vi "RemoteTester.vi"() -> ()   [LabVIEW 2019]
uses:
  <vilib>/Platform/TimedLoop/XDataNode/timing_clust.ctl
  <vilib>/Platform/TimedLoop/XDataNode/nitl_modes.ctl
  <vilib>/Platform/TimedLoop/XDataNode/wakeup.ctl
  <vilib>/myRIO/Instrument Drivers/Onboard IO/DIO/typedefs/DIO Reference.ctl
  <vilib>/myRIO/Common/Instrument Driver Framework/Utilities/typedefs/myRIO Generic Hardware Reference.ctl
  <vilib>/myRIO/Common/Instrument Driver Framework/Utilities/typedefs/Hardware Version Enum.ctl
  <vilib>/myRIO/Common/Instrument Driver Framework/Utilities/typedefs/myRIO v1.0 Reference.ctl
  <vilib>/myRIO/Common/Instrument Driver Framework/Utilities/typedefs/Generic FPGA Reference.ctl
  <vilib>/myRIO/Common/Instrument Driver Framework/myRIO v1.0/DIO/typedefs/DIO Channels List.ctl
  <vilib>/myRIO/Common/Instrument Driver Framework/myRIO v1.0/DIO/typedefs/DIO Channels Enum.ctl
  <vilib>/userDefined/High Color/nirio_resource_hc.ctl
  <vilib>/myRIO/Common/Instrument Driver Framework/Utilities/vis/Is FPGA Ref Available.vi
  <vilib>/myRIO/Common/Instrument Driver Framework/myRIO v1.0/DIO/vis/myRIO v1.1 Open DIO.vi
  <vilib>/myRIO/Instrument Drivers/Onboard IO/DIO/vis/Write.vi
  <vilib>/myRIO/Common/Instrument Driver Framework/Utilities/vis/Validate Channels.vi
  <vilib>/myRIO/Common/Instrument Driver Framework/myRIO v1.0/DIO/vis/myRIO v1.0 Reserve DIO.vi
  <vilib>/myRIO/Common/Instrument Driver Framework/myRIO v1.0/Resource Manager/vis/myRIO v1.0 Reserve Channel List.vi
  <vilib>/myRIO/Common/Instrument Driver Framework/myRIO v1.0/DIO/vis/myRIO v1.0 Build MUX Configuration DIO.vi
  <vilib>/myRIO/Common/Instrument Driver Framework/myRIO v1.0/Resource Manager/vis/myRIO v1.0 Reserve Channel.vi
  <vilib>/myRIO/Common/Instrument Driver Framework/myRIO v1.0/Resource Manager/vis/myRIO v1.0 Unreserve Channel.vi
  <vilib>/myRIO/Common/Instrument Driver Framework/myRIO v1.0/Resource Manager/vis/myRIO v1.0 Create Configuration List.vi
  <vilib>/myRIO/Common/Instrument Driver Framework/myRIO v1.0/Resource Manager/vis/myRIO v1.0 Build Mutex Name.vi
  <vilib>/rvi/Analysis/host/Private/Sample Rate To Loop Time (ticks).vi
  <vilib>/Utility/error.llb/Error Cluster From Error Code.vi
  <vilib>/rvi/errors/niLvFpgaAdjustHostInterfaceError.vi
  <vilib>/measure/mamon.llb/Trigger Detection for 1 Channel.vi
  <vilib>/measure/matone.llb/Extract Single Tone Information 1 Chan.vi
  <vilib>/FPGAPlugInAG/Dynamic/niLvFpga_Abort_Dynamic.vi
  <vilib>/FPGAPlugInAG/Dynamic/niLvFpga_Close_Dynamic.vi
  <vilib>/Utility/VariantDataType/GetNumericInfo.vi
  <vilib>/myRIO/Common/Instrument Driver Framework/myRIO v1.0/myRIO v1.1 Open.vi
  <vilib>/myRIO/Common/Instrument Driver Framework/Utilities/vis/IO Manager.vi
  <vilib>/myRIO/Common/Instrument Driver Framework/Utilities/vis/Configuration Manager.vi
  <vilib>/myRIO/Common/Instrument Driver Framework/myRIO v1.0/Resource Manager/vis/myRIO v1.0 Configure IO.vi
  <vilib>/myRIO/Common/Instrument Driver Framework/myRIO v1.0/myRIO v1.0 Close.vi
  <vilib>/myRIO/Common/Instrument Driver Framework/myRIO v1.0/DIO/vis/myRIO v1.0 Write DIO.vi
  <vilib>/rvi/interface/nirviMethod/nirviMethod.xnode
  <vilib>/rvi/interface/nirviReadWriteControl/nirviReadWriteControl.xnode
  <vilib>/rvi/interface/nirviCloseFPGA/nirviCloseFPGA.xnode
  <vilib>/platform/TimedLoop/XDataNode/XDataNode.xnode
  <vilib>/myRIO/Express VI/Onboard Devices/LED/LED Express VI.xnode
  <vilib>/myRIO/Instrument Drivers/Onboard IO/DIO/vis/myRIO DIO Open.xnode
  <vilib>/rvi/errors/niLvFpgaMergeErrorWithErrorCode.vi
  <vilib>/rvi/interface/Simulation/niFpgaSimulationCallBeginRW.vi
  NiFpgaLv.dll
  <vilib>/rvi/Analysis/host/Public/NI_FpgaMspHost.lvlib
  <vilib>/FPGAPlugInAG/Dynamic/niLvFpga_ReadFifo_Dynamic.vi
  <vilib>/measure/NI_MAPro.lvlib
  <vilib>/Platform/TimedLoop/XDataNode/XDNodeRunTimeDep.lvlib
  <vilib>/myRIO/Instrument Drivers/Onboard IO/DIO/DIO.lvlib
panel:
  out "aLL":dbl[][](array[numeric])
  in  "LED0":bool
  in  "stop test loop":bool
  out "x-y":dbl=43.60094893016756
  out "Freq":dbl=99.99999999997463
  out "G [um/mA]":dbl=0.0002339690708833829 format="%#_2g"
  in  "stop":bool=TRUE
  in  "MainTab":T1(tab)=enum."Bode Analysis"
  in  "Sine wave properties":T2={"Frequency (periods/tick)"=0.0, "Phase offset (periods)"=0.0, "Scale factor"=0.5, "Amplitude offset"=0.0}
  in  "Sampling Rate":dbl=1024.0 max=100000.0
  in  "Generated Frequency(Hz)":dbl=2000.0
  in  "TimeDataTab":enum32{"Output", "Input", "Triggered Data"}(tab)=enum."Triggered Data"
  out "Output Time Data":dbl[](graph)=[2.0856, 2.0856, 2.0823, 2.0856, 2.0823, 2.0856, 2.0823, 2.0856, 2.0856, 2.0823, 2.0856, 2.0823, 2.0856, 2.0823, 2.0856, 2.0823, 2.0823, 2.0856, 2.0823, 2.0823, 2.0823, 2.0856, 2.0856, 2.0823, 2.0856, 2.0823, 2.0856, 2.0856, 2.0856, 2.0823, 2.0856, 2.0856, 2.0856, 2.0856, 2.0856, 2.0856, 2.0823, 2.0856, 2.0856, 2.0823, 2.0856, 2.0856, 2.0823, 2.0823, 2.0856, 2.0823, 2.0823, 2.0856, 2.0856, 2.0856, 2.0823, 2.0856, 2.0823, 2.0823, 2.0856, 2.0856, 2.0856, 2.0823, 2.0889, 2.0856, 2.0856, 2.0856, 2.0856, 2.0856, 2.0823, 2.0823, 2.0823, 2.0823, 2.0856, 2.0823, 2.0856, 2.079, 2.0856, 2.0823, 2.0823, 2.0856, 2.0823, 2.0823, 2.0823, 2.0856, 2.0823, 2.0856, 2.0856, 2.0856, 2.0856, 2.0823, 2.0856, 2.0823, 2.0856, 2.0856, 2.0823, 2.0856, 2.0823, 2.0856, 2.0823, 2.0856, 2.0856, 2.0823, 2.0856, 2.0856, 2.0856, 2.0823, 2.0856, 2.0856, 2.0823, 2.0856, 2.0856, 2.0856, 2.0823, 2.0856, 2.0856, 2.0856, 2.0856, 2.0856, 2.0856, 2.0823, 2.0856, 2.0889, 2.0823, 2.0856, 2.0823, 2.0856, 2.0823, 2.0856, 2.0856, 2.0823, 2.0856, 2.0823, 2.0856, 2.0823, 2.0856, 2.0823, 2.0823, 2.0856, 2.0823, 2.0856, 2.0823, 2.0856, 2.0856, 2.0856, 2.0856, 2.0823, 2.0856, 2.0823, 2.0856, 2.0823, 2.0856, 2.0856, 2.0823, 2.0856, 2.0856, 2.0856, 2.079, 2.0823, 2.0856, 2.0823, 2.0856, 2.0856, 2.0856, 2.0823, 2.0856, 2.0856, 2.0823, 2.0856, 2.0856, 2.0856, 2.0823, 2.0856, 2.0823, 2.0823, 2.0856, 2.0856, 2.0823, 2.079, 2.0889, 2.0823, 2.0823, 2.0856, 2.0823, 2.0823, 2.0823, 2.0856, 2.0856, 2.0823, 2.0856, 2.0856, 2.0823, 2.0823, 2.0856, 2.0823, 2.0823, 2.0823, 2.0856, 2.0823, 2.079, 2.0889, 2.0823, 2.0823, 2.0856, 2.0856, 2.0823, 2.0823, 2.0856, 2.0823, 2.0823, 2.0856, 2.0856, 2.0856, 2.0823, 2.0889, 2.0856, 2.0856, 2.0856, 2.0856, 2.0856, 2.0823, 2.0823, 2.0823, 2.0823, 2.0856, 2.0823, 2.0856, 2.0823, 2.0856, 2.0823, 2.0889, 2.0823, 2.0823, 2.0856, 2.0823, 2.0823, 2.0823, 2.0889, 2.0823, 2.0823, 2.0889, 2.0823, 2.0856, 2.0823, 2.0889, 2.0856, 2.0856, 2.0889, 2.0823, 2.0823, 2.0823, 2.0856, 2.0823, 2.0823, 2.0823, 2.0856, 2.0823, 2.0823, 2.0856, 2.0823, 2.0823, 2.0856, 2.0823, 2.0823, 2.0823, 2.0889, 2.0823, 2.0823, 2.0856, 2.0856, 2.0856, 2.0823, 2.0856, 2.0823, 2.0856, 2.0856, 2.0823, 2.0823, 2.0856, 2.0856, 2.0823, 2.0823, 2.0856, 2.0823, 2.0856, 2.0823, 2.0856, 2.0823, 2.0856, 2.0856, 2.0823, 2.0856, 2.0823, 2.0856, 2.0856, 2.0823, 2.0856, 2.0856, 2.0856, 2.0856, 2.0856, 2.0823, 2.0856, 2.0823, 2.0823, 2.0856, 2.0823, 2.0856, 2.0823, 2.0856, 2.0823, 2.0823, 2.0856, 2.0823, 2.0823, 2.0823, 2.0856, 2.0823, 2.0856, 2.0856, 2.0856, 2.0823, 2.0823, 2.0889, 2.0823, 2.0823, 2.0856, 2.0856, 2.0823, 2.079, 2.0856, 2.0823, 2.079, 2.0856, 2.0823, 2.0856, 2.079, 2.0856, 2.0823, 2.0823, 2.0823, 2.0856, 2.0856, 2.0856, 2.0889, 2.0823, 2.0856, 2.0856, 2.0856, 2.0823, 2.0823, 2.0856, 2.0823, 2.0856, 2.0823, 2.0856, 2.0823, 2.0823, 2.0856, 2.0823, 2.0856, 2.0823, 2.0856, 2.0856, 2.0823, 2.0856, 2.079, 2.0856, 2.0823, 2.0856, 2.0823, 2.0823, 2.0856, 2.0823, 2.0856, 2.0856, 2.0823, 2.0856, 2.0823, 2.0856, 2.079, 2.0889, 2.0823, 2.0823, 2.0823, 2.0823, 2.0823, 2.0823, 2.0856, 2.079, 2.0856, 2.0823, 2.0823, 2.0856, 2.0823, 2.0856, 2.0823, 2.0823, 2.0856, 2.0823, 2.0856, 2.0856, 2.0856, 2.0856, 2.0856, 2.0856, 2.0823, 2.0856, 2.0823, 2.0889, 2.0823, 2.0889, 2.0856, 2.0823, 2.0856, 2.0823, 2.0823, 2.0823, 2.0856, 2.0823, 2.0823, 2.0889, 2.0823, 2.0889, 2.0823, 2.0856, 2.0823, 2.0823, 2.0856, 2.0823, 2.0856, 2.0823, 2.0856, 2.0823, 2.0823, 2.0856, 2.0823, 2.0823, 2.0823, 2.0856, 2.0823, 2.0856, 2.0856, 2.0856, 2.0823, 2.0856, 2.0856, 2.0823, 2.0823, 2.0856, 2.0823, 2.0823, 2.0823, 2.0856, 2.0823, 2.0856, 2.0823, 2.0823, 2.0823, 2.0823, 2.0856, 2.079, 2.0856, 2.0856, 2.0823, 2.0856, 2.0856, 2.0856, 2.0823, 2.0856, 2.0856, 2.0823, 2.0856, 2.0856, 2.0856, 2.0823, 2.0856, 2.0856, 2.0823, 2.079, 2.0856, 2.0856, 2.0823, 2.0856, 2.0856, 2.0856, 2.0856, 2.0823, 2.0889, 2.0823, 2.0856, 2.0856, 2.0823, 2.0856, 2.0823, 2.0856, 2.079, 2.0856, 2.0823, 2.0823, 2.0856, 2.0856, 2.0823, 2.079, 2.0823, 2.0823, 2.0823, 2.0856, 2.0823, 2.0823, 2.0823, 2.0856, 2.0823, 2.0823, 2.0823, 2.0856, 2.0823, 2.0823, 2.0823, 2.0823, 2.0856, 2.0856, 2.0856, 2.0856, 2.0856, 2.0856, 2.0823, 2.0856, 2.0856, 2.0823, 2.0856, 2.0856, 2.0889, 2.0823, 2.0889, 2.0856, 2.0823, 2.0856, 2.0856, 2.0823, 2.079, 2.0856, 2.0856, 2.0823, 2.0856, 2.0856, 2.0856, 2.079, 2.0889, 2.0823, 2.0856, 2.0856, 2.0856, 2.0856, 2.079, 2.0889, 2.0856, 2.0856, 2.0856, 2.0856, 2.0856, 2.079, 2.0889, 2.079, 2.0823, 2.0856, 2.0856, 2.0823, 2.0823, 2.0889, 2.0823, 2.0823, 2.0856, 2.0823, 2.0823, 2.0823, 2.0856, 2.0823, 2.0823, 2.0856, 2.0823, 2.0856, 2.0823, 2.0856, 2.0823, 2.0823, 2.0856, 2.0823, 2.0856, 2.0823, 2.0889, 2.079, 2.0823, 2.0856, 2.0823, 2.0856, 2.0856, 2.0889, 2.0823, 2.0856, 2.0856, 2.0823, 2.0823, 2.0823, 2.0856, 2.079, 2.0856, 2.0856, 2.0856, 2.0823, 2.0823, 2.0856, 2.0823, 2.0856, 2.0823, 2.0856, 2.0823, 2.0823, 2.0856, 2.0856, 2.0889, 2.0823, 2.0856, 2.0856, 2.0823, 2.0823, 2.0823, 2.0856, 2.0823, 2.0856, 2.0856, 2.0823, 2.0856, 2.0823, 2.0856, 2.079, 2.0856, 2.0856, 2.0823, 2.0856, 2.0823, 2.0856, 2.0823, 2.0823, 2.0856, 2.0823, 2.0889, 2.0823, 2.0856, 2.0823, 2.0856, 2.0856, 2.0823, 2.0856, 2.0823, 2.0856, 2.0823, 2.0856, 2.0856, 2.0823, 2.0856, 2.0856, 2.0856, 2.0823, 2.0856, 2.0856, 2.0823, 2.0856, 2.0856, 2.0889, 2.0823, 2.0856, 2.0856, 2.0823, 2.0823, 2.0856, 2.0856, 2.079, 2.0856, 2.0856, 2.0823, 2.0856, 2.0823, 2.0856, 2.0823, 2.0856, 2.079, 2.0856, 2.0856, 2.0823, 2.0856, 2.0823, 2.0856, 2.0823, 2.0823, 2.0856, 2.0823, 2.0823, 2.0823, 2.0856, 2.0823, 2.0856, 2.0856, 2.0823, 2.0856, 2.0823, 2.0856, 2.0823, 2.0856, 2.0856, 2.0823, 2.0823, 2.0856, 2.0889, 2.0823, 2.0856, 2.0889, 2.0823, 2.0856, 2.0823, 2.0856, 2.0823, 2.0856, 2.0889, 2.0823, 2.0856, 2.0823, 2.0889, 2.0823, 2.0856, 2.0856, 2.0823, 2.0823, 2.0856, 2.0856, 2.079, 2.0856, 2.0856, 2.0856, 2.0823, 2.0823, 2.0823, 2.0856, 2.0856, 2.0856, 2.0856, 2.0856, 2.0856, 2.0856, 2.0856, 2.0856, 2.0823, 2.0823, 2.0856, 2.0823, 2.0823, 2.0823, 2.0856, 2.079, 2.0823, 2.0856, 2.0823, 2.0823, 2.0823, 2.0889, 2.079, 2.0856, 2.0856, 2.0823, 2.0823, 2.0823, 2.0889, 2.079, 2.0823, 2.0856, 2.0823, 2.0856, 2.0856, 2.0889, 2.0823, 2.0856, 2.0856, 2.0823, 2.0856, 2.0823, 2.0856, 2.0823, 2.0856, 2.0823, 2.0856, 2.0856, 2.0823, 2.0889, 2.0823, 2.0856, 2.0823, 2.0823, 2.0856, 2.0823, 2.0856, 2.0823, 2.0823, 2.0823, 2.0823, 2.0856, 2.0856, 2.0823, 2.0823, 2.0856, 2.0823, 2.0823, 2.0856, 2.079, 2.0823, 2.0823, 2.0856, 2.0823, 2.0823, 2.0856, 2.0856, 2.0823, 2.0823, 2.0856, 2.0823, 2.0823, 2.0856, 2.0856, 2.0856, 2.0823, 2.0889, 2.0823, 2.0823, 2.0823, 2.0856, 2.0856, 2.0856, 2.0889, 2.0823, 2.0856, 2.0823, 2.0856, 2.0823, 2.0856, 2.0856, 2.0823, 2.0856, 2.0856, 2.0856, 2.0823, 2.0823, 2.0856, 2.0823, 2.0856, 2.0823, 2.0823, 2.0823, 2.0823, 2.0889, 2.0823, 2.0856, 2.0823, 2.0856, 2.0823, 2.0823, 2.0856, 2.0823, 2.0856, 2.0823, 2.0823, 2.0823, 2.0823, 2.0856, 2.0856, 2.0856, 2.0823, 2.0823, 2.0856, 2.0823, 2.0856, 2.0823, 2.0856, 2.0823, 2.0889, 2.0856, 2.0823, 2.0823, 2.0823, 2.0856, 2.079, 2.0856, 2.0856, 2.0823, 2.0856, 2.0856, 2.0856, 2.079, 2.0823, 2.0856, 2.0823, 2.0823, 2.0856, 2.0856, 2.0823, 2.0889, 2.0856, 2.0823, 2.0823, 2.0856, 2.0856, 2.0823, 2.0889, 2.0856, 2.0856, 2.0856, 2.0823, 2.0856, 2.0823, 2.0856, 2.0856, 2.0823, 2.0856, 2.0856, 2.0856, 2.0823, 2.0856, 2.0856, 2.0823, 2.0856, 2.0823, 2.0856, 2.0823, 2.0856, 2.0823, 2.079, 2.0856, 2.0823, 2.0856, 2.0823, 2.0889, 2.0823, 2.0856, 2.0823, 2.0823, 2.0856, 2.0823, 2.0856, 2.079, 2.0856, 2.0856, 2.0823, 2.0856, 2.0823, 2.0856, 2.0823, 2.0856, 2.0856, 2.0823, 2.0856, 2.0856, 2.0856, 2.0856, 2.0856, 2.0856, 2.079, 2.0856, 2.0823, 2.0856, 2.079, 2.0856, 2.0889, 2.0856, 2.0856, 2.0823, 2.0856, 2.079, 2.0856, 2.0856, 2.0823, 2.0856, 2.0856, 2.0889, 2.0823, 2.0856, 2.0823, 2.0823, 2.0856, 2.0823, 2.0856, 2.0823, 2.0856, 2.0856, 2.0856, 2.0856, 2.0823, 2.0823, 2.0823, 2.0856, 2.0823, 2.0823, 2.0856, 2.0823, 2.0823, 2.0823, 2.0856, 2.079, 2.0823, 2.0856, 2.0856, 2.0823, 2.079, 2.0856, 2.0823, 2.0823, 2.0856, 2.0823, 2.0856, 2.0856, 2.0889, 2.0856, 2.0856, 2.0856, 2.0823, 2.0823, 2.0823, 2.0856, 2.0823, 2.0856, 2.0856, 2.0856]
  out "InputTimeData":dbl[](graph)=[6.5538, 6.7485, 6.6594, 6.3096, 5.7222, 4.8609, 3.9567, 3.0294, 2.1252, 1.2012, 0.5808, 0.165, 0.0, 0.132, 0.5148, 1.1088, 2.0097, 2.904, 3.8544, 4.7487, 5.6496, 6.2436, 6.6297, 6.7584, 6.5868, 6.1776, 5.5572, 4.6331999999999995, 3.729, 2.7786, 1.8975, 1.0197, 0.4488, 0.0957, 0.009899999999999999, 0.2112, 0.6534, 1.3002, 2.2407, 3.1515, 4.0986, 5.082, 5.8278, 6.369, 6.6857999999999995, 6.7386, 6.5076, 6.0324, 5.3592, 4.4022, 3.4848, 2.5377, 1.5708, 0.8481, 0.3333, 0.0495, 0.0363, 0.297, 0.8052, 1.6071, 2.4783, 3.399, 4.3395, 5.2932, 5.9928, 6.4746, 6.7254, 6.699, 6.4086, 5.8674, 5.0424, 4.158, 3.234, 2.3199, 1.3662, 0.6897, 0.2343, 0.0165, 0.0825, 0.4092, 0.9768, 1.8215999999999999, 2.7192, 3.6498, 4.5573, 5.4912, 6.1314, 6.567, 6.7584, 6.6462, 6.2898, 5.6958, 4.8246, 3.9138, 2.9865, 2.0856, 1.1715, 0.5577, 0.1518, 0.0, 0.1452, 0.5346, 1.1418, 2.046, 2.9634, 3.894, 4.785, 5.6793, 6.2667, 6.6396, 6.7551, 6.5736, 6.1545, 5.5241999999999996, 4.5936, 3.6894, 2.739, 1.7489999999999999, 0.99, 0.429, 0.0858, 0.0132, 0.2244, 0.6798, 1.3332, 2.2803, 3.1944, 4.1382, 5.115, 5.8542, 6.3888, 6.699, 6.732, 6.4845, 6.006, 5.2041, 4.3626, 3.4419, 2.4981, 1.5378, 0.8184, 0.31679999999999997, 0.0429, 0.0429, 0.31679999999999997, 0.8316, 1.6434, 2.5179, 3.4419, 4.3824, 5.3262, 6.0192, 6.4944, 6.732, 6.6924, 6.3888, 5.841, 5.0094, 4.1184, 3.1944, 2.2605, 1.3332, 0.6666, 0.2178, 0.0033, 0.0924, 0.429, 1.0032, 1.8612, 2.7588, 3.6894, 4.5936, 5.5241999999999996, 6.1545, 6.5802, 6.7584, 6.6363, 6.2667, 5.6628, 4.785, 3.8742, 2.9436, 1.914, 1.1418, 0.5346, 0.1386, 0.0, 0.15839999999999999, 0.5577, 1.188, 2.0856, 3.0063, 3.9369, 4.9533, 5.709, 6.2898, 6.6528, 6.7518, 6.5604, 6.1314, 5.4912, 4.5573, 3.6498, 2.6994, 1.6962, 0.9603, 0.4092, 0.07919999999999999, 0.0165, 0.2409, 0.7029, 1.485, 2.3199, 3.234, 4.1778, 5.1513, 5.8806, 6.4086, 6.7056, 6.7254, 6.468, 5.9796, 5.1678, 4.3197, 3.399, 2.4585, 1.5015, 0.792, 0.297, 0.0363, 0.0495, 0.3333, 0.8613, 1.6962, 2.5575, 3.4848, 4.4187, 5.3592, 6.0456, 6.5076, 6.7518, 6.6857999999999995, 6.369, 5.8145999999999995, 4.9698, 4.0788, 3.1515, 2.2209, 1.3002, 0.6402, 0.2046, 0.0, 0.099, 0.4488, 1.0362, 1.8975, 2.8017, 3.729, 4.7652, 5.5572, 6.1908, 6.5934, 6.7584, 6.6264, 6.2436, 5.6331, 4.7487, 3.8346, 2.904, 1.8777, 1.1088, 0.5148, 0.1287, 0.0, 0.1716, 0.5808, 1.221, 2.1252, 3.0492, 3.9798, 4.9896, 5.7387, 6.3096, 6.6627, 6.7485, 6.5472, 6.1049999999999995, 5.3427, 4.5177, 3.5871, 2.6598, 1.6599, 0.9306, 0.3894, 0.0693, 0.019799999999999998, 0.2574, 0.726, 1.518, 2.3562, 3.2736, 4.2207, 5.1876, 5.9103, 6.4251, 6.732, 6.7221, 6.4515, 5.9532, 5.1348, 4.2801, 3.3594, 2.4189, 1.4652, 0.7656, 0.2838, 0.0132, 0.0594, 0.363, 0.891, 1.7292, 2.6004, 3.5244, 4.4583, 5.3922, 6.0687, 6.5241, 6.7518, 6.6759, 6.3492, 5.7816, 4.9368, 4.0392, 3.1086, 2.0658, 1.2671999999999999, 0.6171, 0.1914, 0.0, 0.1122, 0.4686, 1.0626, 1.9338, 2.8446, 3.7719, 4.8048, 5.5869, 6.2106, 6.6066, 6.7584, 6.6132, 6.2238, 5.6034, 4.7124, 3.795, 2.8644, 1.8414, 1.0791, 0.49169999999999997, 0.1188, 0.0066, 0.1848, 0.6039, 1.3497, 2.1648, 3.0888, 4.0194, 5.0292, 5.7684, 6.3294, 6.6726, 6.7452, 6.534, 6.0786, 5.3064, 4.4781, 3.5442, 2.6202, 1.6236, 0.9042, 0.3696, 0.039599999999999996, 0.0264, 0.2739, 0.7524, 1.5543, 2.3958, 3.3165, 4.2603, 5.2404, 5.94, 6.4416, 6.7353, 6.7155, 6.435, 5.9268, 5.0985, 4.2405, 3.3165, 2.376, 1.4322, 0.7392, 0.264, 0.0132, 0.066, 0.3795, 0.9174, 1.7688, 2.64, 3.564, 4.6134, 5.4252, 6.0918, 6.5405999999999995, 6.7551, 6.666, 6.3294, 5.7552, 4.8807, 3.9996, 3.069, 2.0295, 1.2342, 0.594, 0.1782, 0.0, 0.1221, 0.49169999999999997, 1.188, 1.9734, 2.8842, 3.8148, 4.8444, 5.6166, 6.2337, 6.6198, 6.7584, 6.6, 6.2007, 5.4747, 4.6728, 3.7521, 2.8215, 1.8051, 1.0493999999999999, 0.462, 0.1056, 0.0066, 0.198, 0.627, 1.3827, 2.2011, 3.1284, 4.059, 5.0622, 5.7981, 6.3492, 6.7056, 6.7419, 6.5175, 6.0555, 5.2734, 4.4385, 3.5046, 2.5806, 1.5906, 0.8778, 0.3498, 0.033, 0.033, 0.2904, 0.7788, 1.5906, 2.4387, 3.3792, 4.2999, 5.2734, 5.9664, 6.4614, 6.7386, 6.7089, 6.4152, 5.8971, 5.0622, 4.2009, 3.2736, 2.2209, 1.3992, 0.7128, 0.2508, 0.0066, 0.0726, 0.3993, 0.9438, 1.8051, 2.6796, 3.6069, 4.653, 5.4582, 6.1182, 6.5538, 6.7584, 6.6594, 6.2964, 5.6331, 4.8444, 3.9567, 3.0294, 1.9932, 1.2012, 0.5676, 0.165, 0.0, 0.132, 0.5148, 1.221, 2.0097, 2.9238, 3.8544, 4.8807, 5.6496, 6.2568, 6.6297, 6.7551, 6.5868, 6.1776, 5.4417, 4.6331999999999995, 3.7092, 2.7786, 1.7688, 1.0197, 0.4389, 0.0693, 0.0132, 0.2112, 0.6534, 1.4157, 2.2407, 3.1713, 4.0986, 5.0985, 5.8278, 6.369, 6.7122, 6.7353, 6.501, 6.0324, 5.2404, 4.4022, 3.4617, 2.4189, 1.5543, 0.8481, 0.3333, 0.0264, 0.0363, 0.3069, 0.8052, 1.6236, 2.4783, 3.4188, 4.4583, 5.3064, 5.9928, 6.4746, 6.7452, 6.699, 6.3953999999999995, 5.8674, 5.0292, 4.158, 3.234, 2.1846, 1.3497, 0.6897, 0.2343, 0.0066, 0.0825, 0.4191, 1.0626, 1.8414, 2.7192, 3.6498, 4.6926, 5.4912, 6.1413, 6.567, 6.7584, 6.6462, 6.2766, 5.6034, 4.8048, 3.9138, 2.9865, 1.9536, 1.1715, 0.5478, 0.1518, 0.0, 0.1452, 0.5346, 1.254, 2.0658, 2.9634, 3.894, 4.917, 5.6793, 6.2766, 6.6726, 6.7518, 6.5736, 6.1545, 5.4087, 4.5936, 3.6696, 2.739, 1.7292, 0.99, 0.4191, 0.0594, 0.0132, 0.2244, 0.6798, 1.452, 2.2803, 3.2142, 4.2603, 5.1348, 5.8542, 6.3953999999999995, 6.7188, 6.732, 6.4845, 6.006, 5.2041, 4.3626, 3.4188, 2.376, 1.518, 0.8184, 0.31679999999999997, 0.0231, 0.0429, 0.3234, 0.8316, 1.6599, 2.5179, 3.4617, 4.4979, 5.3427, 6.0192, 6.4944, 6.7452, 6.6924, 6.3789, 5.7552, 4.9896, 4.1184, 3.1713, 2.145, 1.3167, 0.6666, 0.2178, 0.0033, 0.0924, 0.4389, 1.0956, 1.8777, 2.7588, 3.6894, 4.7289, 5.5241999999999996, 6.1644, 6.6264, 6.7584, 6.6363, 6.2568, 5.5704, 4.7652, 3.8742, 2.9436, 1.914, 1.1418, 0.5246999999999999, 0.1056, 0.0, 0.15839999999999999, 0.5676, 1.2837, 2.1054, 3.0063, 3.9369, 4.9533, 5.709, 6.2964, 6.6792, 6.7518, 6.5604, 6.1314, 5.3757, 4.5573, 3.63, 2.5575, 1.6962, 0.9603, 0.3993, 0.0528, 0.019799999999999998, 0.2409, 0.7029, 1.485, 2.3199, 3.2538, 4.2999, 5.1678, 5.8806, 6.4152, 6.7254, 6.7254, 6.468, 5.9796, 5.1678, 4.3197, 3.3792, 2.3397, 1.485, 0.792, 0.297, 0.019799999999999998, 0.0528, 0.3432, 0.9603, 1.6962, 2.5575, 3.5046, 4.5375, 5.3757, 6.0456, 6.5076, 6.7518, 6.6857999999999995, 6.3591, 5.7222, 4.9533, 4.0788, 3.1284, 2.1054, 1.2837, 0.6402, 0.15839999999999999, 0.0, 0.099, 0.462, 1.1253, 1.914, 2.8017, 3.729, 4.7652, 5.5704, 6.1908, 6.6363, 6.7584, 6.6264, 6.2337, 5.5374, 4.7289, 3.8346, 2.904, 1.8777, 1.1088, 0.5016, 0.0957, 0.0033, 0.1716, 0.594, 1.3167, 2.145, 3.0492, 4.1184, 4.9896, 5.7387, 6.3195, 6.6891, 6.7452, 6.5472, 6.1049999999999995, 5.3427, 4.4979, 3.5871, 2.5179, 1.6599, 0.9306, 0.3795, 0.0462, 0.0231, 0.2574, 0.8184, 1.518, 2.3562, 3.2967, 4.3395, 5.2041, 5.9103, 6.435, 6.732, 6.7188, 6.4515, 5.8542, 5.1348, 4.2801, 3.3396, 2.3001, 1.452, 0.7656, 0.2739, 0.0132, 0.0594, 0.363, 0.99, 1.7292, 2.6004, 3.5442, 4.5738, 5.4087, 6.0687, 6.5736, 6.7518, 6.6759, 6.3393, 5.6958, 4.917, 4.0392, 3.0888, 2.0658, 1.254, 0.6171, 0.1452, 0.0, 0.1122, 0.4818, 1.155, 1.9536, 2.8446, 3.795, 4.8048, 5.6034, 6.2106, 6.6462, 6.7584, 6.6132, 6.2106, 5.5044, 4.6926, 3.795, 2.7192, 1.8414, 1.0791, 0.4818, 0.0825, 0.0066, 0.1848, 0.6171, 1.3497, 2.1846, 3.0888, 4.158, 5.0292, 5.7684, 6.3393, 6.699, 6.7452, 6.534, 5.9928, 5.3064, 4.4583, 3.5442, 2.4783, 1.6236, 0.9042, 0.363, 0.039599999999999996, 0.0264, 0.2739, 0.8481, 1.5543, 2.3958, 3.3396, 4.4022, 5.2404, 5.94, 6.4515, 6.7353, 6.7122, 6.435, 5.8278, 5.0985, 4.2405, 3.2967, 2.2605, 1.4157, 0.7392, 0.2112, 0.0132, 0.0693, 0.3795, 1.0197, 1.7688, 2.64, 3.5871, 4.6134, 5.4417, 6.0918, 6.5868, 6.7551, 6.666, 6.3195, 5.6496, 4.8807, 3.9996, 2.9238, 2.0295, 1.221, 0.594, 0.132, 0.0, 0.1221, 0.5016, 1.188, 1.9932, 2.8842, 3.9567, 4.8444, 5.6331, 6.2337, 6.6594, 6.7584, 6.6, 6.1908, 5.4747, 4.653, 3.7521, 2.6796, 1.8051, 1.0362, 0.462, 0.0726, 0.0066, 0.198, 0.7128, 1.3827, 2.2209, 3.1284, 4.2009, 5.0622, 5.7981, 6.3591, 6.7056, 6.7386, 6.5175, 5.9664, 5.2734, 4.4187, 3.5046, 2.4387, 1.5906, 0.8778, 0.3432, 0.033, 0.033, 0.2904, 0.8778, 1.5906, 2.4585, 3.3792, 4.4385, 5.2734, 5.9664, 6.5175, 6.7386, 6.7056, 6.4152, 5.7981, 5.0622, 4.2009, 3.2538, 2.2209, 1.3827, 0.7128, 0.198, 0.0066, 0.07919999999999999, 0.3993, 1.0493999999999999, 1.8051, 2.6796, 3.7521, 4.653, 5.4747, 6.1182, 6.6, 6.7584, 6.6528, 6.2964, 5.6166, 4.8444, 3.9567, 2.8842, 1.9932, 1.188, 0.5676, 0.1221, 0.0, 0.132, 0.5246999999999999, 1.221, 2.0295, 2.9238, 3.9996, 4.8807, 5.6628, 6.2568, 6.666, 6.7551]
  out "Waveform Graph 2":dbl[][](graph)=[[2.0097, 2.904, 3.8544, 4.7487, 5.6496, 6.2436, 6.6297, 6.7584, 6.5868, 6.1776, 5.5572, 4.6331999999999995, 3.729, 2.7786, 1.8975, 1.0197, 0.4488, 0.0957, 0.009899999999999999, 0.2112, 0.6534, 1.3002, 2.2407, 3.1515, 4.0986, 5.082, 5.8278, 6.369, 6.6857999999999995, 6.7386, 6.5076, 6.0324, 5.3592, 4.4022, 3.4848, 2.5377, 1.5708, 0.8481, 0.3333, 0.0495, 0.0363, 0.297, 0.8052, 1.6071, 2.4783, 3.399, 4.3395, 5.2932, 5.9928, 6.4746, 6.7254, 6.699, 6.4086, 5.8674, 5.0424, 4.158, 3.234, 2.3199, 1.3662, 0.6897, 0.2343, 0.0165, 0.0825, 0.4092, 0.9768, 1.8215999999999999, 2.7192, 3.6498, 4.5573, 5.4912, 6.1314, 6.567, 6.7584, 6.6462, 6.2898, 5.6958, 4.8246, 3.9138, 2.9865, 2.0856, 1.1715, 0.5577, 0.1518, 0.0, 0.1452, 0.5346, 1.1418, 2.046, 2.9634, 3.894, 4.785, 5.6793, 6.2667, 6.6396, 6.7551, 6.5736, 6.1545, 5.5241999999999996, 4.5936, 3.6894, 2.739, 1.7489999999999999, 0.99, 0.429, 0.0858, 0.0132, 0.2244, 0.6798, 1.3332, 2.2803, 3.1944, 4.1382, 5.115, 5.8542, 6.3888, 6.699, 6.732, 6.4845, 6.006, 5.2041, 4.3626, 3.4419, 2.4981, 1.5378, 0.8184, 0.31679999999999997, 0.0429, 0.0429, 0.31679999999999997, 0.8316, 1.6434, 2.5179, 3.4419, 4.3824, 5.3262, 6.0192, 6.4944, 6.732, 6.6924, 6.3888, 5.841, 5.0094, 4.1184, 3.1944, 2.2605, 1.3332, 0.6666, 0.2178, 0.0033, 0.0924, 0.429, 1.0032, 1.8612, 2.7588, 3.6894, 4.5936, 5.5241999999999996, 6.1545, 6.5802, 6.7584, 6.6363, 6.2667, 5.6628, 4.785, 3.8742, 2.9436, 1.914, 1.1418, 0.5346, 0.1386, 0.0, 0.15839999999999999, 0.5577, 1.188, 2.0856, 3.0063, 3.9369, 4.9533, 5.709, 6.2898, 6.6528, 6.7518, 6.5604, 6.1314, 5.4912, 4.5573, 3.6498, 2.6994, 1.6962, 0.9603, 0.4092, 0.07919999999999999, 0.0165, 0.2409, 0.7029, 1.485, 2.3199, 3.234, 4.1778, 5.1513, 5.8806, 6.4086, 6.7056, 6.7254, 6.468, 5.9796, 5.1678, 4.3197, 3.399, 2.4585, 1.5015, 0.792, 0.297, 0.0363, 0.0495, 0.3333, 0.8613, 1.6962, 2.5575, 3.4848, 4.4187, 5.3592, 6.0456, 6.5076, 6.7518, 6.6857999999999995, 6.369, 5.8145999999999995, 4.9698, 4.0788, 3.1515, 2.2209, 1.3002, 0.6402, 0.2046, 0.0, 0.099, 0.4488, 1.0362, 1.8975, 2.8017, 3.729, 4.7652, 5.5572, 6.1908, 6.5934, 6.7584, 6.6264, 6.2436, 5.6331, 4.7487, 3.8346, 2.904, 1.8777, 1.1088, 0.5148, 0.1287, 0.0, 0.1716, 0.5808, 1.221, 2.1252, 3.0492, 3.9798, 4.9896, 5.7387, 6.3096, 6.6627, 6.7485, 6.5472, 6.1049999999999995, 5.3427, 4.5177, 3.5871, 2.6598, 1.6599, 0.9306, 0.3894, 0.0693, 0.019799999999999998, 0.2574, 0.726, 1.518, 2.3562, 3.2736, 4.2207, 5.1876, 5.9103, 6.4251, 6.732, 6.7221, 6.4515, 5.9532, 5.1348, 4.2801, 3.3594, 2.4189, 1.4652, 0.7656, 0.2838, 0.0132, 0.0594, 0.363, 0.891, 1.7292, 2.6004, 3.5244, 4.4583, 5.3922, 6.0687, 6.5241, 6.7518, 6.6759, 6.3492, 5.7816, 4.9368, 4.0392, 3.1086, 2.0658, 1.2671999999999999, 0.6171, 0.1914, 0.0, 0.1122, 0.4686, 1.0626, 1.9338, 2.8446, 3.7719, 4.8048, 5.5869, 6.2106, 6.6066, 6.7584, 6.6132, 6.2238, 5.6034, 4.7124, 3.795, 2.8644, 1.8414, 1.0791, 0.49169999999999997, 0.1188, 0.0066, 0.1848, 0.6039, 1.3497, 2.1648, 3.0888, 4.0194, 5.0292, 5.7684, 6.3294, 6.6726, 6.7452, 6.534, 6.0786, 5.3064, 4.4781, 3.5442, 2.6202, 1.6236, 0.9042, 0.3696, 0.039599999999999996, 0.0264, 0.2739, 0.7524, 1.5543, 2.3958, 3.3165, 4.2603, 5.2404, 5.94, 6.4416, 6.7353, 6.7155, 6.435, 5.9268, 5.0985, 4.2405, 3.3165, 2.376, 1.4322, 0.7392, 0.264, 0.0132, 0.066, 0.3795, 0.9174, 1.7688, 2.64, 3.564, 4.6134, 5.4252, 6.0918, 6.5405999999999995, 6.7551, 6.666, 6.3294, 5.7552, 4.8807, 3.9996, 3.069, 2.0295, 1.2342, 0.594, 0.1782, 0.0, 0.1221, 0.49169999999999997, 1.188, 1.9734, 2.8842, 3.8148, 4.8444, 5.6166, 6.2337, 6.6198, 6.7584, 6.6, 6.2007, 5.4747, 4.6728, 3.7521, 2.8215, 1.8051, 1.0493999999999999, 0.462, 0.1056, 0.0066, 0.198, 0.627, 1.3827, 2.2011, 3.1284, 4.059, 5.0622, 5.7981, 6.3492, 6.7056, 6.7419, 6.5175, 6.0555, 5.2734, 4.4385, 3.5046, 2.5806, 1.5906, 0.8778, 0.3498, 0.033, 0.033, 0.2904, 0.7788, 1.5906, 2.4387, 3.3792, 4.2999, 5.2734, 5.9664, 6.4614, 6.7386, 6.7089, 6.4152, 5.8971, 5.0622, 4.2009, 3.2736, 2.2209, 1.3992, 0.7128, 0.2508, 0.0066, 0.0726, 0.3993, 0.9438, 1.8051, 2.6796, 3.6069, 4.653, 5.4582, 6.1182, 6.5538, 6.7584, 6.6594, 6.2964, 5.6331, 4.8444, 3.9567, 3.0294, 1.9932, 1.2012, 0.5676, 0.165, 0.0, 0.132, 0.5148, 1.221, 2.0097, 2.9238, 3.8544, 4.8807, 5.6496, 6.2568, 6.6297, 6.7551, 6.5868, 6.1776, 5.4417, 4.6331999999999995, 3.7092, 2.7786, 1.7688, 1.0197, 0.4389, 0.0693, 0.0132, 0.2112, 0.6534, 1.4157, 2.2407, 3.1713, 4.0986, 5.0985, 5.8278, 6.369, 6.7122, 6.7353, 6.501, 6.0324, 5.2404, 4.4022, 3.4617, 2.4189, 1.5543, 0.8481, 0.3333, 0.0264, 0.0363, 0.3069, 0.8052, 1.6236, 2.4783, 3.4188, 4.4583, 5.3064, 5.9928, 6.4746, 6.7452, 6.699, 6.3953999999999995, 5.8674, 5.0292, 4.158, 3.234, 2.1846, 1.3497, 0.6897, 0.2343, 0.0066, 0.0825, 0.4191, 1.0626, 1.8414, 2.7192, 3.6498, 4.6926, 5.4912, 6.1413, 6.567, 6.7584, 6.6462, 6.2766, 5.6034, 4.8048, 3.9138, 2.9865, 1.9536, 1.1715, 0.5478, 0.1518, 0.0, 0.1452, 0.5346, 1.254, 2.0658, 2.9634, 3.894, 4.917, 5.6793, 6.2766, 6.6726, 6.7518, 6.5736, 6.1545, 5.4087, 4.5936, 3.6696, 2.739, 1.7292, 0.99, 0.4191, 0.0594, 0.0132, 0.2244, 0.6798, 1.452, 2.2803, 3.2142, 4.2603, 5.1348, 5.8542, 6.3953999999999995, 6.7188, 6.732, 6.4845, 6.006, 5.2041, 4.3626, 3.4188, 2.376, 1.518, 0.8184, 0.31679999999999997, 0.0231, 0.0429, 0.3234, 0.8316, 1.6599, 2.5179, 3.4617, 4.4979, 5.3427, 6.0192, 6.4944, 6.7452, 6.6924, 6.3789, 5.7552, 4.9896, 4.1184, 3.1713, 2.145, 1.3167, 0.6666, 0.2178, 0.0033, 0.0924, 0.4389, 1.0956, 1.8777, 2.7588, 3.6894, 4.7289, 5.5241999999999996, 6.1644, 6.6264, 6.7584, 6.6363, 6.2568, 5.5704, 4.7652, 3.8742, 2.9436, 1.914, 1.1418, 0.5246999999999999, 0.1056, 0.0, 0.15839999999999999, 0.5676, 1.2837, 2.1054, 3.0063, 3.9369, 4.9533, 5.709, 6.2964, 6.6792, 6.7518, 6.5604, 6.1314, 5.3757, 4.5573, 3.63, 2.5575, 1.6962, 0.9603, 0.3993, 0.0528, 0.019799999999999998, 0.2409, 0.7029, 1.485, 2.3199, 3.2538, 4.2999, 5.1678, 5.8806, 6.4152, 6.7254, 6.7254, 6.468, 5.9796, 5.1678, 4.3197, 3.3792, 2.3397, 1.485, 0.792, 0.297, 0.019799999999999998, 0.0528, 0.3432, 0.9603, 1.6962, 2.5575, 3.5046, 4.5375, 5.3757, 6.0456, 6.5076, 6.7518, 6.6857999999999995, 6.3591, 5.7222, 4.9533, 4.0788, 3.1284, 2.1054, 1.2837, 0.6402, 0.15839999999999999, 0.0, 0.099, 0.462, 1.1253, 1.914, 2.8017, 3.729, 4.7652, 5.5704, 6.1908, 6.6363, 6.7584, 6.6264, 6.2337, 5.5374, 4.7289, 3.8346, 2.904, 1.8777, 1.1088, 0.5016, 0.0957, 0.0033, 0.1716, 0.594, 1.3167, 2.145, 3.0492, 4.1184, 4.9896, 5.7387, 6.3195, 6.6891, 6.7452, 6.5472, 6.1049999999999995, 5.3427, 4.4979, 3.5871, 2.5179, 1.6599, 0.9306, 0.3795, 0.0462, 0.0231, 0.2574, 0.8184, 1.518, 2.3562, 3.2967, 4.3395, 5.2041, 5.9103, 6.435, 6.732, 6.7188, 6.4515, 5.8542, 5.1348, 4.2801, 3.3396, 2.3001, 1.452, 0.7656, 0.2739, 0.0132, 0.0594, 0.363, 0.99, 1.7292, 2.6004, 3.5442, 4.5738, 5.4087, 6.0687, 6.5736, 6.7518, 6.6759, 6.3393, 5.6958, 4.917, 4.0392, 3.0888, 2.0658, 1.254, 0.6171, 0.1452, 0.0, 0.1122, 0.4818, 1.155, 1.9536, 2.8446, 3.795, 4.8048, 5.6034, 6.2106, 6.6462, 6.7584, 6.6132, 6.2106, 5.5044, 4.6926, 3.795, 2.7192, 1.8414, 1.0791, 0.4818, 0.0825, 0.0066, 0.1848, 0.6171, 1.3497, 2.1846, 3.0888, 4.158, 5.0292, 5.7684, 6.3393, 6.699, 6.7452, 6.534, 5.9928, 5.3064, 4.4583, 3.5442, 2.4783, 1.6236, 0.9042, 0.363, 0.039599999999999996, 0.0264, 0.2739, 0.8481, 1.5543, 2.3958, 3.3396, 4.4022, 5.2404, 5.94, 6.4515, 6.7353, 6.7122, 6.435, 5.8278, 5.0985, 4.2405, 3.2967, 2.2605, 1.4157, 0.7392, 0.2112, 0.0132, 0.0693, 0.3795, 1.0197, 1.7688, 2.64, 3.5871, 4.6134, 5.4417, 6.0918, 6.5868, 6.7551, 6.666, 6.3195, 5.6496, 4.8807, 3.9996, 2.9238, 2.0295, 1.221, 0.594, 0.132, 0.0, 0.1221, 0.5016, 1.188, 1.9932, 2.8842, 3.9567, 4.8444, 5.6331, 6.2337, 6.6594, 6.7584, 6.6, 6.1908, 5.4747, 4.653, 3.7521, 2.6796, 1.8051, 1.0362, 0.462, 0.0726, 0.0066, 0.198, 0.7128, 1.3827, 2.2209, 3.1284, 4.2009, 5.0622, 5.7981, 6.3591, 6.7056, 6.7386, 6.5175, 5.9664, 5.2734, 4.4187, 3.5046, 2.4387, 1.5906, 0.8778, 0.3432, 0.033, 0.033, 0.2904, 0.8778, 1.5906, 2.4585, 3.3792, 4.4385, 5.2734, 5.9664, 6.5175, 6.7386, 6.7056, 6.4152, 5.7981, 5.0622, 4.2009, 3.2538, 2.2209, 1.3827, 0.7128, 0.198, 0.0066, 0.07919999999999999, 0.3993, 1.0493999999999999, 1.8051, 2.6796, 3.7521, 4.653, 5.4747, 6.1182, 6.6, 6.7584, 6.6528, 6.2964, 5.6166, 4.8444, 3.9567, 2.8842, 1.9932, 1.188, 0.5676, 0.1221, 0.0, 0.132, 0.5246999999999999, 1.221, 2.0295, 2.9238, 3.9996, 4.8807, 5.6628, 6.2568, 6.666, 6.7551], [2.0823, 2.0856, 2.0823, 2.0823, 2.0823, 2.0856, 2.0856, 2.0823, 2.0856, 2.0823, 2.0856, 2.0856, 2.0856, 2.0823, 2.0856, 2.0856, 2.0856, 2.0856, 2.0856, 2.0856, 2.0823, 2.0856, 2.0856, 2.0823, 2.0856, 2.0856, 2.0823, 2.0823, 2.0856, 2.0823, 2.0823, 2.0856, 2.0856, 2.0856, 2.0823, 2.0856, 2.0823, 2.0823, 2.0856, 2.0856, 2.0856, 2.0823, 2.0889, 2.0856, 2.0856, 2.0856, 2.0856, 2.0856, 2.0823, 2.0823, 2.0823, 2.0823, 2.0856, 2.0823, 2.0856, 2.079, 2.0856, 2.0823, 2.0823, 2.0856, 2.0823, 2.0823, 2.0823, 2.0856, 2.0823, 2.0856, 2.0856, 2.0856, 2.0856, 2.0823, 2.0856, 2.0823, 2.0856, 2.0856, 2.0823, 2.0856, 2.0823, 2.0856, 2.0823, 2.0856, 2.0856, 2.0823, 2.0856, 2.0856, 2.0856, 2.0823, 2.0856, 2.0856, 2.0823, 2.0856, 2.0856, 2.0856, 2.0823, 2.0856, 2.0856, 2.0856, 2.0856, 2.0856, 2.0856, 2.0823, 2.0856, 2.0889, 2.0823, 2.0856, 2.0823, 2.0856, 2.0823, 2.0856, 2.0856, 2.0823, 2.0856, 2.0823, 2.0856, 2.0823, 2.0856, 2.0823, 2.0823, 2.0856, 2.0823, 2.0856, 2.0823, 2.0856, 2.0856, 2.0856, 2.0856, 2.0823, 2.0856, 2.0823, 2.0856, 2.0823, 2.0856, 2.0856, 2.0823, 2.0856, 2.0856, 2.0856, 2.079, 2.0823, 2.0856, 2.0823, 2.0856, 2.0856, 2.0856, 2.0823, 2.0856, 2.0856, 2.0823, 2.0856, 2.0856, 2.0856, 2.0823, 2.0856, 2.0823, 2.0823, 2.0856, 2.0856, 2.0823, 2.079, 2.0889, 2.0823, 2.0823, 2.0856, 2.0823, 2.0823, 2.0823, 2.0856, 2.0856, 2.0823, 2.0856, 2.0856, 2.0823, 2.0823, 2.0856, 2.0823, 2.0823, 2.0823, 2.0856, 2.0823, 2.079, 2.0889, 2.0823, 2.0823, 2.0856, 2.0856, 2.0823, 2.0823, 2.0856, 2.0823, 2.0823, 2.0856, 2.0856, 2.0856, 2.0823, 2.0889, 2.0856, 2.0856, 2.0856, 2.0856, 2.0856, 2.0823, 2.0823, 2.0823, 2.0823, 2.0856, 2.0823, 2.0856, 2.0823, 2.0856, 2.0823, 2.0889, 2.0823, 2.0823, 2.0856, 2.0823, 2.0823, 2.0823, 2.0889, 2.0823, 2.0823, 2.0889, 2.0823, 2.0856, 2.0823, 2.0889, 2.0856, 2.0856, 2.0889, 2.0823, 2.0823, 2.0823, 2.0856, 2.0823, 2.0823, 2.0823, 2.0856, 2.0823, 2.0823, 2.0856, 2.0823, 2.0823, 2.0856, 2.0823, 2.0823, 2.0823, 2.0889, 2.0823, 2.0823, 2.0856, 2.0856, 2.0856, 2.0823, 2.0856, 2.0823, 2.0856, 2.0856, 2.0823, 2.0823, 2.0856, 2.0856, 2.0823, 2.0823, 2.0856, 2.0823, 2.0856, 2.0823, 2.0856, 2.0823, 2.0856, 2.0856, 2.0823, 2.0856, 2.0823, 2.0856, 2.0856, 2.0823, 2.0856, 2.0856, 2.0856, 2.0856, 2.0856, 2.0823, 2.0856, 2.0823, 2.0823, 2.0856, 2.0823, 2.0856, 2.0823, 2.0856, 2.0823, 2.0823, 2.0856, 2.0823, 2.0823, 2.0823, 2.0856, 2.0823, 2.0856, 2.0856, 2.0856, 2.0823, 2.0823, 2.0889, 2.0823, 2.0823, 2.0856, 2.0856, 2.0823, 2.079, 2.0856, 2.0823, 2.079, 2.0856, 2.0823, 2.0856, 2.079, 2.0856, 2.0823, 2.0823, 2.0823, 2.0856, 2.0856, 2.0856, 2.0889, 2.0823, 2.0856, 2.0856, 2.0856, 2.0823, 2.0823, 2.0856, 2.0823, 2.0856, 2.0823, 2.0856, 2.0823, 2.0823, 2.0856, 2.0823, 2.0856, 2.0823, 2.0856, 2.0856, 2.0823, 2.0856, 2.079, 2.0856, 2.0823, 2.0856, 2.0823, 2.0823, 2.0856, 2.0823, 2.0856, 2.0856, 2.0823, 2.0856, 2.0823, 2.0856, 2.079, 2.0889, 2.0823, 2.0823, 2.0823, 2.0823, 2.0823, 2.0823, 2.0856, 2.079, 2.0856, 2.0823, 2.0823, 2.0856, 2.0823, 2.0856, 2.0823, 2.0823, 2.0856, 2.0823, 2.0856, 2.0856, 2.0856, 2.0856, 2.0856, 2.0856, 2.0823, 2.0856, 2.0823, 2.0889, 2.0823, 2.0889, 2.0856, 2.0823, 2.0856, 2.0823, 2.0823, 2.0823, 2.0856, 2.0823, 2.0823, 2.0889, 2.0823, 2.0889, 2.0823, 2.0856, 2.0823, 2.0823, 2.0856, 2.0823, 2.0856, 2.0823, 2.0856, 2.0823, 2.0823, 2.0856, 2.0823, 2.0823, 2.0823, 2.0856, 2.0823, 2.0856, 2.0856, 2.0856, 2.0823, 2.0856, 2.0856, 2.0823, 2.0823, 2.0856, 2.0823, 2.0823, 2.0823, 2.0856, 2.0823, 2.0856, 2.0823, 2.0823, 2.0823, 2.0823, 2.0856, 2.079, 2.0856, 2.0856, 2.0823, 2.0856, 2.0856, 2.0856, 2.0823, 2.0856, 2.0856, 2.0823, 2.0856, 2.0856, 2.0856, 2.0823, 2.0856, 2.0856, 2.0823, 2.079, 2.0856, 2.0856, 2.0823, 2.0856, 2.0856, 2.0856, 2.0856, 2.0823, 2.0889, 2.0823, 2.0856, 2.0856, 2.0823, 2.0856, 2.0823, 2.0856, 2.079, 2.0856, 2.0823, 2.0823, 2.0856, 2.0856, 2.0823, 2.079, 2.0823, 2.0823, 2.0823, 2.0856, 2.0823, 2.0823, 2.0823, 2.0856, 2.0823, 2.0823, 2.0823, 2.0856, 2.0823, 2.0823, 2.0823, 2.0823, 2.0856, 2.0856, 2.0856, 2.0856, 2.0856, 2.0856, 2.0823, 2.0856, 2.0856, 2.0823, 2.0856, 2.0856, 2.0889, 2.0823, 2.0889, 2.0856, 2.0823, 2.0856, 2.0856, 2.0823, 2.079, 2.0856, 2.0856, 2.0823, 2.0856, 2.0856, 2.0856, 2.079, 2.0889, 2.0823, 2.0856, 2.0856, 2.0856, 2.0856, 2.079, 2.0889, 2.0856, 2.0856, 2.0856, 2.0856, 2.0856, 2.079, 2.0889, 2.079, 2.0823, 2.0856, 2.0856, 2.0823, 2.0823, 2.0889, 2.0823, 2.0823, 2.0856, 2.0823, 2.0823, 2.0823, 2.0856, 2.0823, 2.0823, 2.0856, 2.0823, 2.0856, 2.0823, 2.0856, 2.0823, 2.0823, 2.0856, 2.0823, 2.0856, 2.0823, 2.0889, 2.079, 2.0823, 2.0856, 2.0823, 2.0856, 2.0856, 2.0889, 2.0823, 2.0856, 2.0856, 2.0823, 2.0823, 2.0823, 2.0856, 2.079, 2.0856, 2.0856, 2.0856, 2.0823, 2.0823, 2.0856, 2.0823, 2.0856, 2.0823, 2.0856, 2.0823, 2.0823, 2.0856, 2.0856, 2.0889, 2.0823, 2.0856, 2.0856, 2.0823, 2.0823, 2.0823, 2.0856, 2.0823, 2.0856, 2.0856, 2.0823, 2.0856, 2.0823, 2.0856, 2.079, 2.0856, 2.0856, 2.0823, 2.0856, 2.0823, 2.0856, 2.0823, 2.0823, 2.0856, 2.0823, 2.0889, 2.0823, 2.0856, 2.0823, 2.0856, 2.0856, 2.0823, 2.0856, 2.0823, 2.0856, 2.0823, 2.0856, 2.0856, 2.0823, 2.0856, 2.0856, 2.0856, 2.0823, 2.0856, 2.0856, 2.0823, 2.0856, 2.0856, 2.0889, 2.0823, 2.0856, 2.0856, 2.0823, 2.0823, 2.0856, 2.0856, 2.079, 2.0856, 2.0856, 2.0823, 2.0856, 2.0823, 2.0856, 2.0823, 2.0856, 2.079, 2.0856, 2.0856, 2.0823, 2.0856, 2.0823, 2.0856, 2.0823, 2.0823, 2.0856, 2.0823, 2.0823, 2.0823, 2.0856, 2.0823, 2.0856, 2.0856, 2.0823, 2.0856, 2.0823, 2.0856, 2.0823, 2.0856, 2.0856, 2.0823, 2.0823, 2.0856, 2.0889, 2.0823, 2.0856, 2.0889, 2.0823, 2.0856, 2.0823, 2.0856, 2.0823, 2.0856, 2.0889, 2.0823, 2.0856, 2.0823, 2.0889, 2.0823, 2.0856, 2.0856, 2.0823, 2.0823, 2.0856, 2.0856, 2.079, 2.0856, 2.0856, 2.0856, 2.0823, 2.0823, 2.0823, 2.0856, 2.0856, 2.0856, 2.0856, 2.0856, 2.0856, 2.0856, 2.0856, 2.0856, 2.0823, 2.0823, 2.0856, 2.0823, 2.0823, 2.0823, 2.0856, 2.079, 2.0823, 2.0856, 2.0823, 2.0823, 2.0823, 2.0889, 2.079, 2.0856, 2.0856, 2.0823, 2.0823, 2.0823, 2.0889, 2.079, 2.0823, 2.0856, 2.0823, 2.0856, 2.0856, 2.0889, 2.0823, 2.0856, 2.0856, 2.0823, 2.0856, 2.0823, 2.0856, 2.0823, 2.0856, 2.0823, 2.0856, 2.0856, 2.0823, 2.0889, 2.0823, 2.0856, 2.0823, 2.0823, 2.0856, 2.0823, 2.0856, 2.0823, 2.0823, 2.0823, 2.0823, 2.0856, 2.0856, 2.0823, 2.0823, 2.0856, 2.0823, 2.0823, 2.0856, 2.079, 2.0823, 2.0823, 2.0856, 2.0823, 2.0823, 2.0856, 2.0856, 2.0823, 2.0823, 2.0856, 2.0823, 2.0823, 2.0856, 2.0856, 2.0856, 2.0823, 2.0889, 2.0823, 2.0823, 2.0823, 2.0856, 2.0856, 2.0856, 2.0889, 2.0823, 2.0856, 2.0823, 2.0856, 2.0823, 2.0856, 2.0856, 2.0823, 2.0856, 2.0856, 2.0856, 2.0823, 2.0823, 2.0856, 2.0823, 2.0856, 2.0823, 2.0823, 2.0823, 2.0823, 2.0889, 2.0823, 2.0856, 2.0823, 2.0856, 2.0823, 2.0823, 2.0856, 2.0823, 2.0856, 2.0823, 2.0823, 2.0823, 2.0823, 2.0856, 2.0856, 2.0856, 2.0823, 2.0823, 2.0856, 2.0823, 2.0856, 2.0823, 2.0856, 2.0823, 2.0889, 2.0856, 2.0823, 2.0823, 2.0823, 2.0856, 2.079, 2.0856, 2.0856, 2.0823, 2.0856, 2.0856, 2.0856, 2.079, 2.0823, 2.0856, 2.0823, 2.0823, 2.0856, 2.0856, 2.0823, 2.0889, 2.0856, 2.0823, 2.0823, 2.0856, 2.0856, 2.0823, 2.0889, 2.0856, 2.0856, 2.0856, 2.0823, 2.0856, 2.0823, 2.0856, 2.0856, 2.0823, 2.0856, 2.0856, 2.0856, 2.0823, 2.0856, 2.0856, 2.0823, 2.0856, 2.0823, 2.0856, 2.0823, 2.0856, 2.0823, 2.079, 2.0856, 2.0823, 2.0856, 2.0823, 2.0889, 2.0823, 2.0856, 2.0823, 2.0823, 2.0856, 2.0823, 2.0856, 2.079, 2.0856, 2.0856, 2.0823, 2.0856, 2.0823, 2.0856, 2.0823, 2.0856, 2.0856, 2.0823, 2.0856, 2.0856, 2.0856, 2.0856, 2.0856, 2.0856, 2.079, 2.0856, 2.0823, 2.0856, 2.079, 2.0856, 2.0889, 2.0856, 2.0856, 2.0823, 2.0856, 2.079, 2.0856, 2.0856, 2.0823, 2.0856, 2.0856, 2.0889, 2.0823, 2.0856, 2.0823, 2.0823, 2.0856, 2.0823, 2.0856, 2.0823, 2.0856, 2.0856, 2.0856, 2.0856, 2.0823, 2.0823, 2.0823, 2.0856, 2.0823, 2.0823, 2.0856, 2.0823, 2.0823, 2.0823, 2.0856, 2.079, 2.0823, 2.0856, 2.0856, 2.0823, 2.079, 2.0856, 2.0823, 2.0823, 2.0856, 2.0823, 2.0856, 2.0856, 2.0889, 2.0856, 2.0856, 2.0856, 2.0823, 2.0823, 2.0823, 2.0856, 2.0823, 2.0856, 2.0856, 2.0856]]
  out "Phase Mismatch":dbl=43.60094893016756
  in  "spectrum type":enum8{"Power (Vrms^2)", "Amplitude (Vrms)"}(ring)=enum."Amplitude (Vrms)"
  out "Fast Fourier Transform":waveform(dbl)(graph)={"t0"=timestamp(0 s since 1904-01-01), "dt"=1.0000128001638422, "Y"=array[512 elements]}
  in  "BodeTab":enum32{"Magnitude", "Phase"}(tab)
  out "Bode Magnitude Plot":waveform(dbl)(graph)={"t0"=timestamp(0 s since 1904-01-01), "dt"=1.0, "Y"=array[30002 elements]}
  out "Bode Phase Plot":waveform(dbl)(graph)={"t0"=timestamp(0 s since 1904-01-01), "dt"=1.0, "Y"=array[30002 elements]}
  in  "Initial Amp":dbl=6.7
  in  "End Freq.":dbl=100.0
  in  "Bode":bool
  in  "Start Frequency":dbl=10.0
  in  "Points/Decade":i32=30000
  out "Elements Remaining":u32
  out "Elements Remaining 2":u32
  out "latest notification":dbl=0.00022765541277286323
  # "Phase"
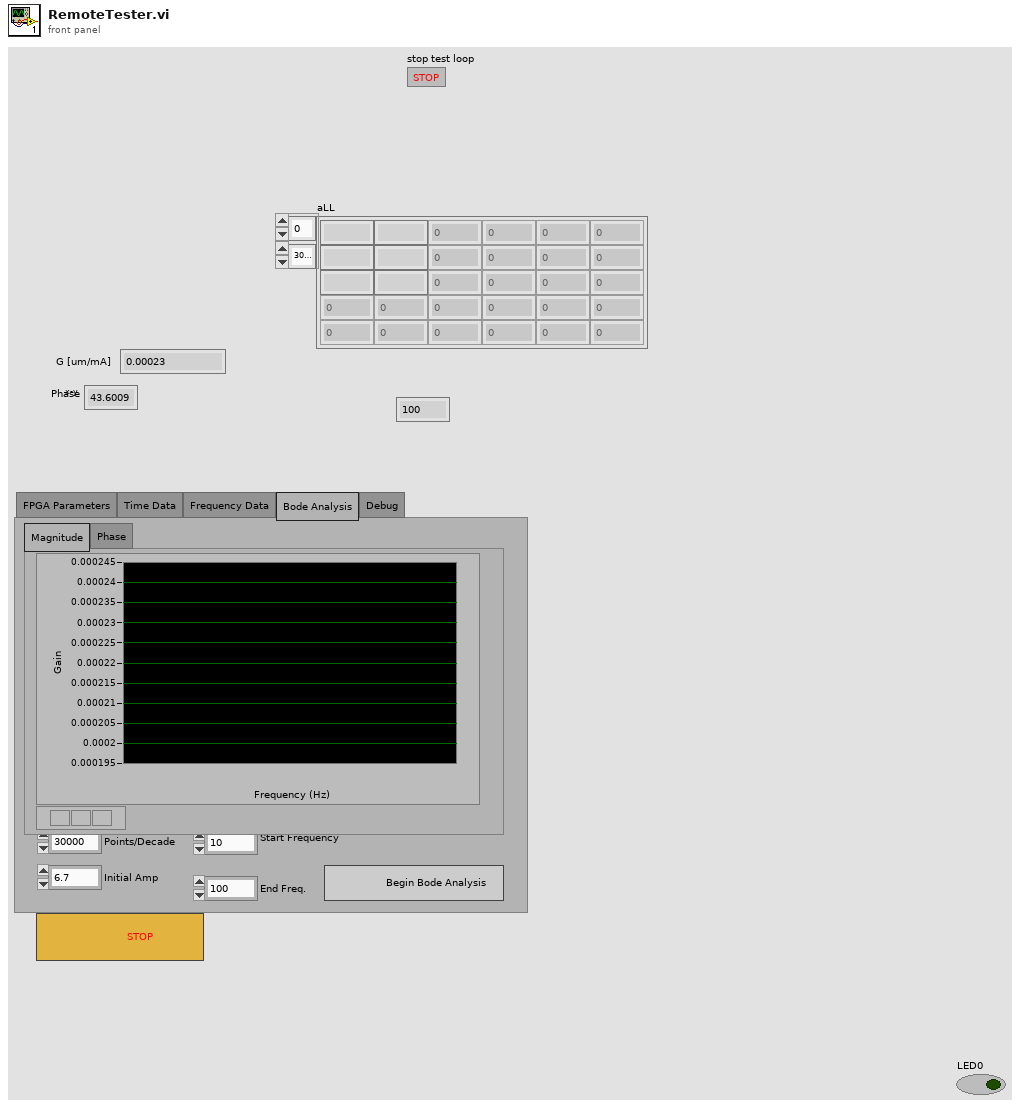
[diagram p1: front panel]
types:
  T1 = enum32{"FPGA Parameters", "Time Data", "Frequency Data", "Bode Analysis", "Debug"}
  T2 = cluster{"Frequency (periods/tick)":fxp<+,32,0>, "Phase offset (periods)":fxp<+,32,0>, "Scale factor":fxp<+,12,1>, "Amplitude offset":fxp<+/-,16,12>}
  T3 = typedef "XDNodeRunTimeDep.lvlib/timing_clust.ctl" = cluster{"Expected End [f-1]":u64, "Actual End [f-1]":u64, "Finished Late? [f-1]":bool, "Expected End [i-1]":u64, "Actual End [i-1]":u64, "Finished Late? [i-1]":bool, "Expected Start [i]":u64, "Actual Start [i]":u64, "Expected Start [f]":u64, "Actual Start [f]":u64, "Source Name":string, "Structure Name":string, "Period":i64, "Deadline":i64, "Offset":i64, "Start":i64, "Priority":i32, "Timeout":i32, "Mode":T4, "Wakeup Reason":T5, "Error":errorcluster, "Source Type":string, "Secondary Source Type":string, "Global End Time":u64, "Global Start Time":u64, "Frame Duration":u64, "Iteration Duration":u64, "Assigned CPU":i32, "I/O Scan Engine Mode":u32}
  T4 = typedef "XDNodeRunTimeDep.lvlib/nitl_modes.ctl" = enum32{"No Change", "Process missed periods, maintain original phase", "Discard missed periods, maintain original phase", "Process missed periods, ignore original phase", "Discard missed periods, ignore original phase"}
  T5 = typedef "XDNodeRunTimeDep.lvlib/wakeup.ctl" = enum32{"Normal", "Aborted", "Asynchronous wakeup", "Timing source error", "Timed loop error", "Timeout"}
  T6 = typedef "DIO.lvlib/DIO Reference.ctl" = cluster{"myRIO Reference":T7, "DIO Channels List":T11}
  T7 = typedef "myRIO Generic Hardware Reference.ctl" = cluster{"myRIO Model":T8, "myRIO Hardware Reference":T9}
  T8 = typedef "Hardware Version Enum.ctl" = enum16{"Unknown", "myRIO-1900", "myRIO-1950", "roboRIO", "NI ELVIS RIO CM", "ELVIS III"}
  T9 = typedef "myRIO v1.0 Reference.ctl" = cluster{"Generic FPGA Reference":T10, "Allow multiple opens":bool}
  T10 = typedef "Generic FPGA Reference.ctl" = refnum<k20>
  T11 = typedef "DIO Channels List.ctl" = T12[]
  T12 = typedef "DIO Channels Enum.ctl" = enum16{"Not Connected", "C/DIO0", "C/DIO1", "C/DIO2", "C/DIO3", "C/DIO4", "C/DIO5", "C/DIO6", "C/DIO7", "A/DIO0", "A/DIO1", "A/DIO2", "A/DIO3", "A/DIO4", "A/DIO5", "A/DIO6", "A/DIO7", "A/DIO8", "A/DIO9", "A/DIO10", "A/DIO11", "A/DIO12", "A/DIO13", "A/DIO14", "A/DIO15", "A/DIO16", "A/DIO17", "A/DIO18", "A/DIO19", "B/DIO0", "B/DIO1", "B/DIO2", "B/DIO3", "B/DIO4", "B/DIO5", "B/DIO6", "B/DIO7", "B/DIO8", "B/DIO9", "B/DIO10", "B/DIO11", "B/DIO12", "B/DIO13", "B/DIO14", "B/DIO15", "B/DIO16", "B/DIO17", "B/DIO18", "B/DIO19", "LED0", "LED1", "LED2", "LED3", "Button0", "DIO/DIO0", "DIO/DIO1", "DIO/DIO2", "DIO/DIO3", "DIO/DIO4", "DIO/DIO5", "DIO/DIO6", "DIO/DIO7", "DIO/DIO8", "DIO/DIO9", "SPI/CS0", "SPI/CS1", "SPI/CS2", "SPI/CS3", "LED RADIO (Green)", "LED RADIO (Red)", "LED COMM (Green)", "LED COMM (Red)", "LED MODE (Green)", "LED MODE (Red)"}
  T13 = typedef "nirio_resource_hc.ctl" = tag
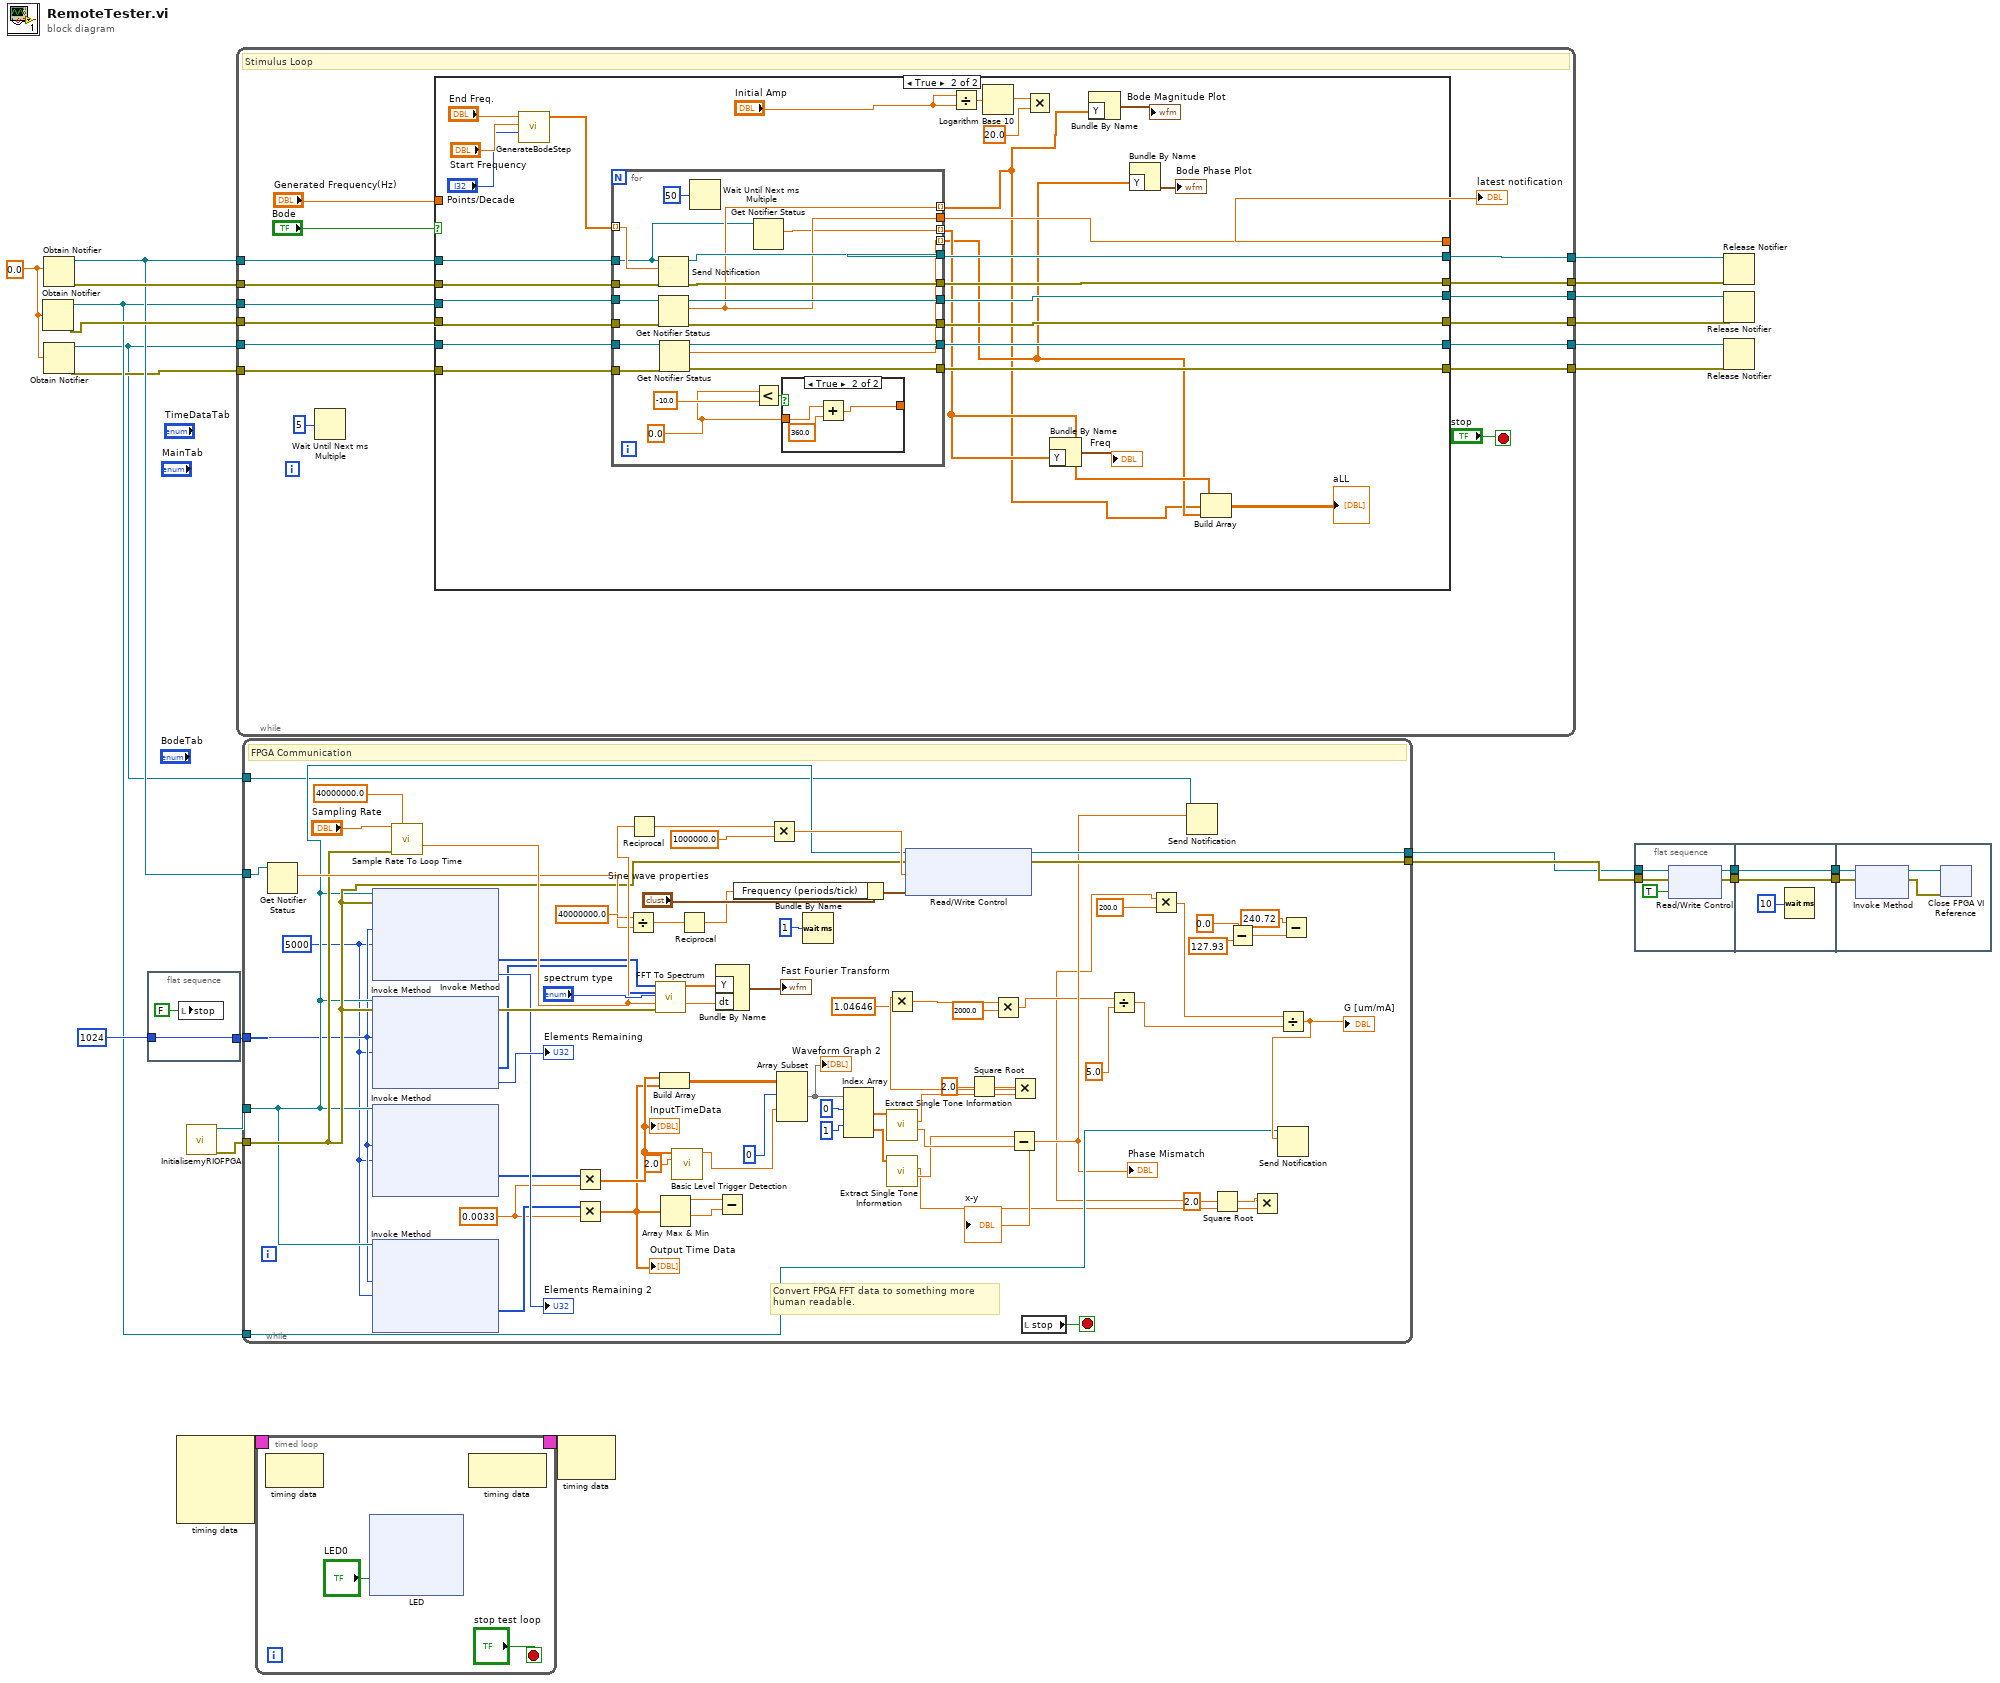
[diagram p0: block diagram]
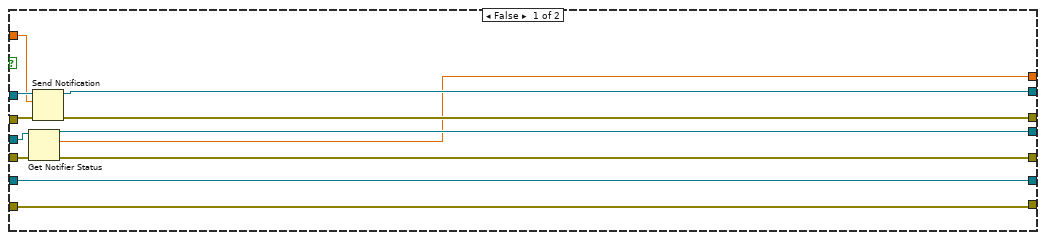
[diagram p2: hidden frame]
diagram:
  w16 = 0.0
  n1 = Obtain Notifier(notification data type=w16) -> (notifier out=w13:refnum<notifier>, error out=w20:errorcluster)  [unwired: 3 in, 1 out]
  n2 = Obtain Notifier(notification data type=w16) -> (notifier out=w15:refnum<notifier>, error out=w23:errorcluster)  [unwired: 3 in, 1 out]
  n3 = Obtain Notifier(notification data type=w16) -> (notifier out=w9:refnum<notifier>, error out=w10:errorcluster)  [unwired: 3 in, 1 out]
  n4 = flat-sequence {
    tunnel: u32 1024 ("Number of Elements") -> [w27]
    tunnel: [w27] -> w14
    frame #0 {
      n5 = local write "stop"(FALSE ("stop")) -> ()
    }
  }
  n6 = node-c288() -> (w2:T3)  [unwired: 4 in]
  n7 = call "InitialisemyRIOFPGA.vi"() -> ("error out"=w11:errorcluster, "Refnum out"=w12:refnum<k20>)  [unwired: 10 in]
  n8 = while {
    tunnel: w15 -> [w44]
    tunnel: w23 -> [w43]
    tunnel: [w42] -> w22
    tunnel: [w41] -> w21
    tunnel: w13 -> [w39]
    tunnel: w20 -> [w38]
    tunnel: [w37] -> w19
    tunnel: [w36] -> w18
    tunnel: w9 -> [w31]
    tunnel: w10 -> [w30]
    tunnel: [w29] -> w8
    tunnel: [w28] -> w7
    stop <- "stop" stop-if-true
    # "Stimulus Loop"
    n9 = Wait Until Next ms Multiple(millisecond multiple=u32 5) -> ()  [unwired: 1 out]
    n10 = case shown="True" "Bode" {
      tunnel: w44 -> [w56 w84]
      tunnel: w43 -> [w55 w81]
      tunnel: [w54 w83] -> w42
      tunnel: [w53 w82] -> w41
      tunnel: w39 -> [w52 w80]
      tunnel: w38 -> [w51 w79]
      tunnel: [w50 w78] -> w37
      tunnel: [w49 w77] -> w36
      tunnel: "Generated Frequency(Hz)" -> [w48 _]
      tunnel: [w47 w76] -> w33
      tunnel: w31 -> [w46 w71]
      tunnel: w30 -> [w45 w70]
      tunnel: [w46 w69] -> w29
      tunnel: [w45 w68] -> w28
      frame False {
        n11 = Get Notifier Status(notifier=w52, error in (no error)=w51) -> (notifier out=w50:refnum<notifier>, current notification=w47:dbl, error out=w49:errorcluster)  [unwired: 2 out]
        n12 = Send Notification(notification=w48, notifier=w56, error in (no error)=w55) -> (notifier out=w54:refnum<notifier>, error out=w53:errorcluster)
      }
      frame True {
        n13 = call "GenerateBodeStep.vi"("Points/Decade"="Points/Decade", "Start Frequency"="Start Frequency", "End Frequency"="End Freq.") -> ("Log-Frequencies"=w63:dbl[])  [unwired: 8 in]
        n14 = for {
          tunnel: w84 -> [w88]
          tunnel: [w104] -> w83
          tunnel: [w103] -> w82
          tunnel: w81 -> [w102]
          tunnel: w80 -> [w101]
          tunnel: w79 -> [w100]
          tunnel: [w99] -> w78
          tunnel: [w98] -> w77
          tunnel: [w96] -> w57 mode=indexing
          tunnel: [w96] -> w76
          tunnel: w71 -> [w95]
          tunnel: w70 -> [w94]
          tunnel: [w93] -> w69
          tunnel: [w92] -> w68
          tunnel: [w86] -> w59 mode=indexing
          tunnel: w63 -> [w90] mode=indexing
          tunnel: [w87] -> w60 mode=indexing
          w85 = 0.0
          n15 = Send Notification(notification=w90, notifier=w88, error in (no error)=w102) -> (notifier out=w104:refnum<notifier>, error out=w103:errorcluster)
          n16 = Get Notifier Status(notifier=w101, error in (no error)=w100) -> (notifier out=w99:refnum<notifier>, current notification=w96:dbl, error out=w98:errorcluster)  [unwired: 2 out]
          n17 = Get Notifier Status(notifier=w95, error in (no error)=w94) -> (notifier out=w93:refnum<notifier>, current notification=w86:dbl, error out=w92:errorcluster)  [unwired: 2 out]
          n18 = Wait Until Next ms Multiple(millisecond multiple=u32 50) -> ()  [unwired: 1 out]
          n19 = Get Notifier Status(notifier=w88) -> (current notification=w87:dbl)  [unwired: 1 in, 4 out]
          n20 = Less?(x=w85, y=-10.0) -> (x < y?=w91:bool)
          n21 = case shown="True" w91 {
            tunnel: w85 -> [w105 w108]
            tunnel: [w105 w106] -> _
            frame False {
            }
            frame True {
              n22 = Add(x=w108, y=360.0) -> (x+y=w106:dbl)
            }
          }
        }
        n23 = Divide(x="Initial Amp", y="Initial Amp") -> (x/y=w74:dbl)
        n24 = Logarithm Base 10(1:w74) -> (0:w73:dbl)
        n25 = Multiply(x=w73, y=20.0) -> ()  [unwired: 1 out]
        n26 = Bundle By Name("Y"=w60) -> (→"Freq":waveform(dbl))  [unwired: 1 in]
        n27 = Bundle By Name("Y"=w57) -> (→"Bode Magnitude Plot":waveform(dbl))  [unwired: 1 in]
        n28 = Bundle By Name("Y"=w59) -> (→"Bode Phase Plot":waveform(dbl))  [unwired: 1 in]
        n29 = Build Array(w60, w57, w59) -> (→"aLL":dbl[][])
      }
    }
    "latest notification" <- w33
  }
  n30 = while {
    tunnel: w12 -> [w140]
    tunnel: w11 -> [w158]
    tunnel: [w137] -> w24
    tunnel: [w136] -> w25
    tunnel: w14 -> [w139]
    tunnel: w15 -> [w157]
    tunnel: w13 -> [w132]
    tunnel: w9 -> [w135]
    stop <- w159 stop-if-true
    w141 = 0.0033
    w138 = 5000 ("Timeout (ms)")
    # "Convert FPGA FFT data to something more\nhuman readable."
    # "FPGA Communication"
    n31 = Get Notifier Status(notifier=w157) -> (current notification=w162:dbl)  [unwired: 1 in, 4 out]
    n32 = xnode "Invoke Method"("FPGA VI Reference In"=w140, "error in"=w158, "Number of Elements"=w139, "Timeout (ms)"=w138) -> ("Data"=w160:i16[], "Elements Remaining"=→"Elements Remaining 2":u32)  [unwired: 2 out]
    n33 = xnode "Invoke Method"("FPGA VI Reference In"=w140, "error in"=w158, "Number of Elements"=w139, "Timeout (ms)"=w138) -> ("error out"=w178:errorcluster, "Data"=w161:i16[], "Elements Remaining"=→"Elements Remaining":u32)  [unwired: 1 out]
    n34 = xnode "Invoke Method"("FPGA VI Reference In"=w140, "Number of Elements"=w139, "Timeout (ms)"=w138) -> ("Data"=w152:i16[])  [unwired: 1 in, 3 out]
    n35 = xnode "Invoke Method"("FPGA VI Reference In"=w140, "Number of Elements"=w139, "Timeout (ms)"=w138) -> ("Data"=w155:i16[])  [unwired: 1 in, 3 out]
    n36 = call-poly <vilib>:"Sample Rate To Loop Time.vi"("sample rate (S/s)"="Sampling Rate", "FPGA clock rate (Hz)"=40000000.0, "error in (no error)"=w158) -> ("actual sample rate (S/s)"=w173:dbl)  [unwired: 10 in, 2 out]
    n37 = Multiply(x=w152, y=w141) -> (x*y=w142:dbl[])
    "InputTimeData" <- w142
    n38 = Multiply(x=w155, y=w141) -> (x*y=w134:dbl[])
    "Output Time Data" <- w134
    n39 = Divide(x=40000000.0 ("FPGA clock rate (Hz)"), y=w162) -> (x/y=w166:dbl)
    n40 = Reciprocal(x=w173) -> (1/x=w170:dbl)
    n41 = call <vilib>:"FFT To Spectrum.vi"("real FFT data"=w160, "imaginary FFT data"=w161, "spectrum type"="spectrum type", "sample rate (S/s)"=w173, "error in (no error)"=w178) -> ("spectrum out"=w177:dbl[], "df (Hz)"=w176:dbl)  [unwired: 8 in, 1 out]
    n42 = Build Array(w142, w134) -> (w143:dbl[][])
    n43 = Array Max & Min(array=w134) -> (max value=w154:dbl, min value=w153:dbl)  [unwired: 2 out]
    n44 = call-poly <vilib>:"Basic Level Trigger Detection.vi"("signal in"=w142, "level"=2.0) -> ("trigger location"=w150:dbl)  [unwired: 11 in, 2 out]
    n45 = Reciprocal(x=w166) -> (1/x=w165:dbl)
    n46 = Bundle By Name("Y"=w177, "dt"=w176) -> (→"Fast Fourier Transform":waveform(dbl))  [unwired: 1 in]
    n47 = Subtract(x=w154, y=w153) -> ()  [unwired: 1 out]
    n48 = Bundle By Name(cluster="Sine wave properties", "Frequency (periods/tick)"=w165) -> (w163:T2)
    n49 = Multiply(x=w170, y=1000000.0) -> (x*y=w168:dbl)
    n50 = Array Subset(array=w143, index (row)=0 ("index"), index (col)=w150) -> (w148:dbl[][])  [unwired: 2 in]
    "Waveform Graph 2" <- w148
    n51 = Wait (ms)(milliseconds to wait=u32 1) -> ()  [unwired: 1 out]
    n52 = Index Array(array=w148, index (row) #1=0 ("index (row)"), index (row) #2=1 ("index (row)")) -> (element #1=w145:dbl[], element #2=w144:dbl[])  [unwired: 2 in]
    n53 = call-poly <vilib>:"Extract Single Tone Information.vi"("time signal in"=w145) -> ("detected phase (deg)"=w130:dbl, "detected amplitude"=w116:dbl)  [unwired: 5 in, 4 out]
    n54 = call-poly <vilib>:"Extract Single Tone Information.vi"("time signal in"=w144) -> ("detected phase (deg)"=w129:dbl, "detected amplitude"=w112:dbl)  [unwired: 5 in, 4 out]
    n55 = xnode "Read/Write Control"("FPGA VI Reference In"=w140, "error in"=w158, "Count(mSec)"=w168, "Sine wave properties"=w163) -> ("FPGA VI Reference Out"=w137:refnum<k20>, "error out"=w136:errorcluster)
    n56 = Square Root(x=2.0) -> (sqrt(x)=w117:dbl)
    n57 = Subtract(x=w129, y=w130) -> (x-y=w131:dbl)
    "Phase Mismatch" <- w131
    "x-y" <- w131
    n58 = Multiply(x=w117, y=w116) -> (x*y=w110:dbl)
    n59 = Multiply(x=w110, y=1.04646) -> (x*y=w111:dbl)
    n60 = Multiply(x=w111, y=2000.0) -> (x*y=w128:dbl)
    n61 = local read "stop"() -> (w159:bool)
    n62 = Divide(x=w128, y=5.0) -> (x/y=w122:dbl)
    n63 = Send Notification(notification=w131, notifier=w135) -> ()  [unwired: 1 in, 2 out]
    n64 = Square Root(x=2.0) -> (sqrt(x)=w114:dbl)
    n65 = Subtract(x=0.0, y=127.93) -> (x-y=w121:dbl)
    n66 = Multiply(x=w114, y=w112) -> (x*y=w113:dbl)
    n67 = Multiply(x=w113, y=200.0) -> (x*y=w120:dbl)
    n68 = Divide(x=w120, y=w122) -> (x/y=w133:dbl)
    "G [um/mA]" <- w133
    n69 = Send Notification(notification=w133, notifier=w132) -> ()  [unwired: 1 in, 2 out]
    n70 = Subtract(x=240.72, y=w121) -> ()  [unwired: 1 out]
  }
  n71 = timed-loop {
    timing: w2 -> [_]
    timing-out: [_] -> w1
    stop <- "stop test loop" stop-if-true
    n72 = node-c288() -> ()  [unwired: 1 in, 1 out]
    n73 = xnode "LED"("LED0"="LED0") -> ()  [unwired: 1 in, 1 out]
    n74 = node-c288() -> ()  [unwired: 1 in, 1 out]
  }
  n75 = node-c288(w1) -> ()  [unwired: 1 out]
  n76 = flat-sequence {
    tunnel: w25 -> [w224]
    tunnel: w24 -> [w223]
    tunnel: [w222] -> w6
    tunnel: [w221] -> w5
    tunnel: w6 -> [w225]
    tunnel: w5 -> [w226]
    tunnel: [w226] -> w4
    tunnel: [w225] -> w3
    tunnel: w4 -> [w229]
    tunnel: w3 -> [w228]
    frame #0 {
      n77 = xnode "Read/Write Control"("FPGA VI Reference In"=w223, "error in"=w224, "stop"=TRUE) -> ("FPGA VI Reference Out"=w221:refnum<k20>, "error out"=w222:errorcluster)
    }
    frame #1 {
      n78 = Wait (ms)(milliseconds to wait=u32 10) -> ()  [unwired: 1 out]
    }
    frame #2 {
      n79 = xnode "Invoke Method"("FPGA VI Reference In"=w229, "error in"=w228) -> ("FPGA VI Reference Out"=w231:refnum<k20>, "error out"=w230:errorcluster)
      n80 = xnode "Close FPGA VI Reference"("FPGA VI Reference In"=w231, "error in"=w230) -> ()  [unwired: 1 out]
    }
  }
  n81 = Release Notifier(notifier=w22, error in (no error)=w21) -> ()  [unwired: 1 in, 3 out]
  n82 = Release Notifier(notifier=w19, error in (no error)=w18) -> ()  [unwired: 1 in, 3 out]
  n83 = Release Notifier(notifier=w8, error in (no error)=w7) -> ()  [unwired: 1 in, 3 out]
